vi "To JSON.vi"(11 "Sequencing Status Value in":refnum<class "Sequencing Status Value.lvclass">) -> (2 "Status JSON":string)   [LabVIEW 2020, in "VolatusSeq.lvlib" / "Sequencing Status Value.lvclass"]
uses:
  Sequencing Status Value.lvclass
  Sequencing Status Value.lvclass/Sequencing Status Value.ctl
  Sequence Status JSON.ctl
  Sequencing Status JSON.ctl
  VolatusSeq.lvlib
  lv-vecto/Vecto/Vecto.lvlib
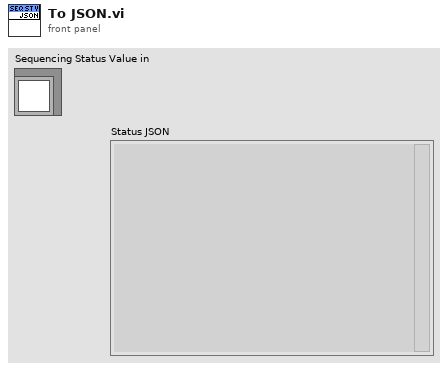
[diagram p1: front panel]
types:
  T1 = typedef "VolatusSeq.lvlib/Sequencing Status JSON.ctl" = cluster{"sequences":T2[]}
  T2 = typedef "VolatusSeq.lvlib/Sequence Status JSON.ctl" = cluster{"name":string, "state":string, "running":bool, "abort":bool, "time":cluster{"seq":i64, "state":i64, "wall":i64}, "loaded":bool, "started":i64, "crc":u32, "color_bg":string, "error":errorcluster, "period":i64, "late":bool}
  T3 = typedef "VolatusSeq.lvlib/Sequencing Status.ctl" = cluster{"Sequences":T4[]}
  T4 = typedef "VolatusSeq.lvlib/Sequence Status Extended.ctl" = cluster{"Status":T5, "Loaded":bool, "CRC32":u32, "BG Color":string, "error":errorcluster}
  T5 = typedef "VolatusSeq.lvlib/Sequence Status.ctl" = cluster{"Name":string, "State":string, "Time":T6, "Running":bool, "Start Time":dbl, "Previous Duration":i64, "Previous Late":bool}
  T6 = typedef "VolatusSeq.lvlib/Sequence Time.ctl" = cluster{"Abort":bool, "Seq Time":dbl, "State Time":dbl, "Wall Time":dbl}
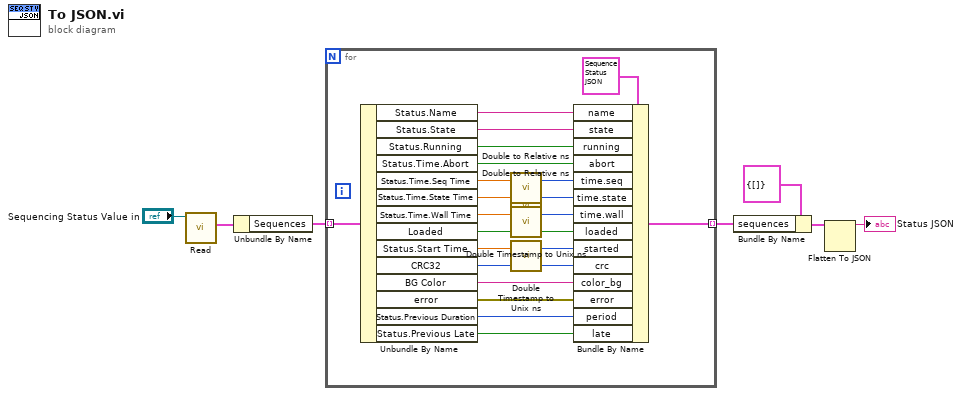
[diagram p0: block diagram]
diagram:
  n1 = call "Read.vi"("Sequencing Status Value in"="Sequencing Status Value in") -> ("Status"=w3:T3)  [unwired: 10 in]
  n2 = Unbundle By Name(w3) -> ("Sequences"=w6:T4[])
  n3 = for {
    tunnel: w6 -> [w28] mode=indexing
    tunnel: [w16] -> w4 mode=indexing
    n4 = Unbundle By Name(w28) -> ("Status.Name"=w26:string, "Status.State"=w25:string, "Status.Running"=w24:bool, "Status.Time.Abort"=w23:bool, "Status.Time.Seq Time"=w22:dbl, "Status.Time.State Time"=w20:dbl, "Status.Time.Wall Time"=w18:dbl, "Loaded"=w15:bool, "Status.Start Time"=w14:dbl, "CRC32"=w12:u32, "BG Color"=w11:string, "error"=w10:errorcluster, "Status.Previous Duration"=w9:i64, "Status.Previous Late"=w8:bool)
    n5 = call "Double to Relative ns.vi"("Double"=w22) -> ("Relative ns"=w21:i64)  [unwired: 2 in]
    n6 = call "Double to Relative ns.vi"("Double"=w20) -> ("Relative ns"=w19:i64)  [unwired: 2 in]
    n7 = call "Double Timestamp to Unix ns.vi"("Timestamp"=w18) -> ("unix ns"=w17:i64)  [unwired: 2 in]
    n8 = call "Double Timestamp to Unix ns.vi"("Timestamp"=w14) -> ("unix ns"=w13:i64)  [unwired: 2 in]
    n9 = Bundle By Name(cluster=T2 {"name"="", "state"="", "running"=FALSE, "abort"=FALSE, "time"={"seq"=0, "state"=0, "wall"=0}, "loaded"=FALSE, "started"=0, "crc"=0, "color_bg"="", "error"={"status"=FALSE, "code"=0, "source"=""}, "period"=0, "late"=FALSE} ("Sequence Status JSON"), "name"=w26, "state"=w25, "running"=w24, "abort"=w23, "time.seq"=w21, "time.state"=w19, "time.wall"=w17, "loaded"=w15, "started"=w13, "crc"=w12, "color_bg"=w11, "error"=w10, "period"=w9, "late"=w8) -> (w16:T2)
  }
  n10 = Bundle By Name(cluster=T1 {"sequences"=[]} ("Sequencing Status JSON"), "sequences"=w4) -> (w2:T1)
  n11 = Flatten To JSON(anything=w2) -> (JSON string=→"Status JSON":string)  [unwired: 2 in, 1 out]
